vi "Cheval_State_Machine.vi"(11 "Cheval_Button":bool) -> (1 "Arm_Defense":T1, 2 "Cheval_Active":bool, 3 "Intake_Pos":T2=enum."Intake Portcullis")   [LabVIEW 2015]
uses:
  Intake Enum..ctl
  Arm_defense_Type_Def.ctl
panel:
  # "Josh Merkle 2/6/16"
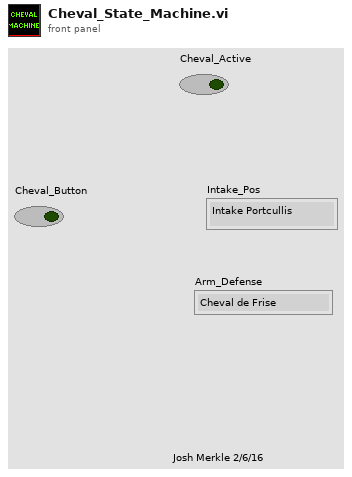
[diagram p1: front panel]
types:
  T1 = typedef "Arm_defense_Type_Def.ctl" = enum16{"Cheval de Frise", "Portcullis", "Out", "In", "Ball_Pickup"}
  T2 = typedef "Intake Enum..ctl" = enum16{"Float", "Intake Portcullis", "Intake Ball Pickup", "Intake Cheval", " Intake Raised"}
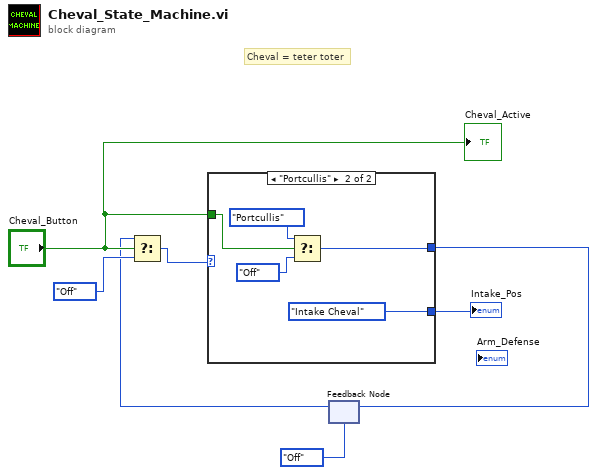
[diagram p0: block diagram]
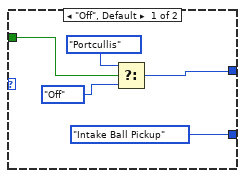
[diagram p2: hidden frame]
diagram:
  # "Cheval = teter toter"
  n1 = feedback #1(enum16{"Off", "Portcullis"}."Off") -> (w4:enum16{"Off", "Portcullis"})
  n2 = Select(t=w4, s="Cheval_Button", f=enum16{"Off", "Portcullis"}."Off") -> (s? t:f=w6:enum16{"Off", "Portcullis"})
  n3 = case shown="\"Portcullis\"" w6 {
    tunnel: "Cheval_Button" -> [w12 w17]
    tunnel: [w9 w14] -> w3
    tunnel: [Intake_Enum.."Intake Ball Pickup" ("Enum") Intake_Enum.."Intake Cheval" ("Enum")] -> w1
    frame "Off", Default {
      n4 = Select(t=enum16{"Off", "Portcullis"}."Portcullis", s=w12, f=enum16{"Off", "Portcullis"}."Off") -> (s? t:f=w9:enum16{"Off", "Portcullis"})
    }
    frame "Portcullis" {
      n5 = Select(t=enum16{"Off", "Portcullis"}."Portcullis", s=w17, f=enum16{"Off", "Portcullis"}."Off") -> (s? t:f=w14:enum16{"Off", "Portcullis"})
    }
  }
  "Intake_Pos" <- w1
  n6 = feedback-in #1(w3) -> ()
  "Cheval_Active" <- "Cheval_Button"
